vi "LcTimer_Init.vi"(0 "reference in":refnum<class "LcTimer.lvclass"> caption="This control should only be used when\na sub class is inheriting this class", 5 "error in (no error)":errorcluster) -> (14 "reference out":refnum<class "LcTimer.lvclass"> caption="This indicator should only be used when\na sub class is inheriting this class", 19 "error out":errorcluster)   [LabVIEW 2020, in "LcTimer.lvclass"]
uses:
  LcTimer.lvclass
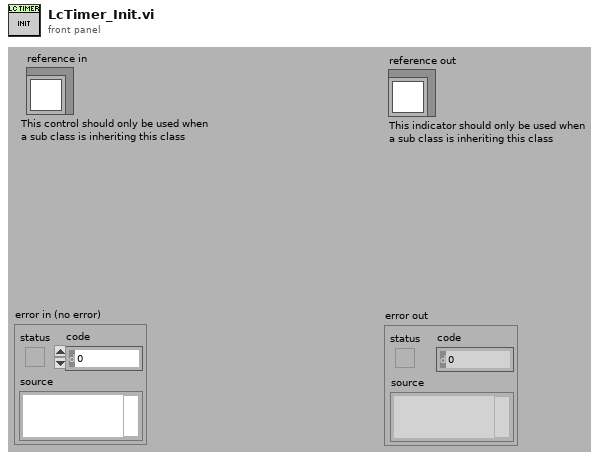
[diagram p1: front panel]
types:
  T1 = typedef "G4BaseTemplate_Singleton_6x8x6.lvclass/ObjectAttributes.ctl" = cluster{"Attribute1":dbl}
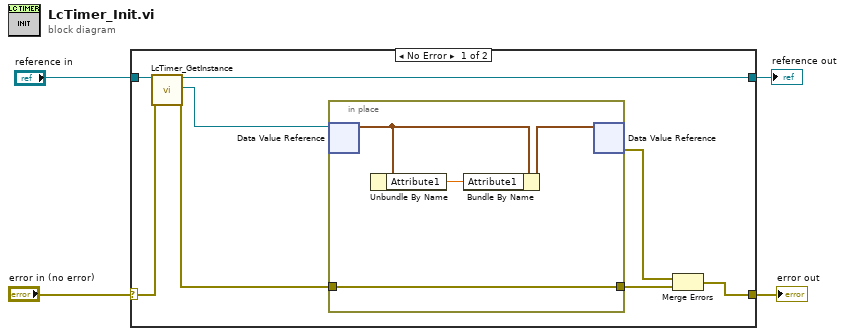
[diagram p0: block diagram]
diagram:
  n1 = case shown="No Error" "error in (no error)" {
    selector: "error in (no error)" -> [w10 w18]
    tunnel: [w11 w18] -> w3
    tunnel: "reference in" -> [w9 w17]
    tunnel: [w8 w17] -> w1
    frame No Error {
      n2 = call "LcTimer_GetInstance.vi"("reference in"=w9, "error in (no error)"=w10) -> ("reference out"=w8:refnum<class "LcTimer.lvclass">, "DVRRefOut"=w7:refnum<data-value>, "error out"=w6:errorcluster)  [unwired: 13 in, 2 out]
      n3 = in-place {
        in-place-border: w6 -> [w13]
        in-place-border: [w13] -> w5
        n4 = in-place-dvr #1(w7) -> (w15:T1)  [unwired: 1 out]
        n5 = Unbundle By Name(w15) -> ("Attribute1"=w14:dbl)
        n6 = Bundle By Name(cluster=w15, "Attribute1"=w14) -> (w16:T1)
        n7 = in-place-dvr #1(w16) -> (w12:errorcluster)  [unwired: 1 out]
      }
      n8 = Merge Errors(w12, w5) -> (w11:errorcluster)
    }
    frame Error {
    }
  }
  "error out" <- w3
  "reference out" <- w1
